vi "Lab_2_subVI_tank_2_Ashish.vi"(0 "H1":dbl, 1 "a1":dbl, 2 "a2":dbl, 3 "A2":dbl, 4 "hss,1":dbl, 5 "hss,2":dbl) -> (14 "H 2":dbl, 15 "h2":dbl)   [LabVIEW 2020]
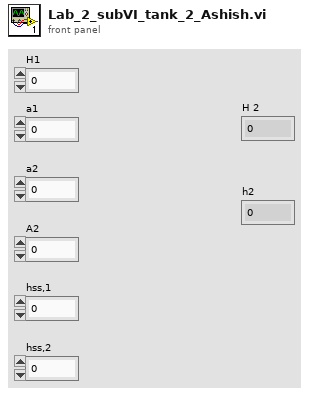
[diagram p1: front panel]
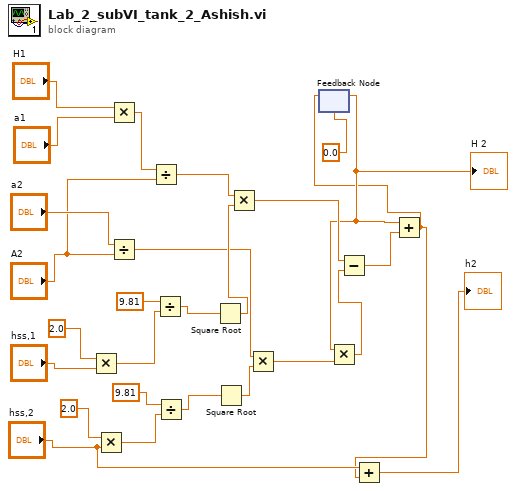
[diagram p0: block diagram]
diagram:
  n1 = Multiply(x=2.0, y="hss,1") -> (x*y=w19:dbl)
  n2 = Multiply(x=2.0, y="hss,2") -> (x*y=w13:dbl)
  n3 = Multiply(x="H1", y="a1") -> (x*y=w24:dbl)
  n4 = Divide(x="a2", y="A2") -> (x/y=w11:dbl)
  n5 = Divide(x=w24, y="A2") -> (x/y=w16:dbl)
  n6 = Divide(x=9.81, y=w19) -> (x/y=w18:dbl)
  n7 = Divide(x=9.81 ("y"), y=w13) -> (x/y=w12:dbl)
  n8 = Square Root(x=w18) -> (sqrt(x)=w17:dbl)
  n9 = Square Root(x=w12) -> (sqrt(x)=w10:dbl)
  n10 = Multiply(x=w16, y=w17) -> (x*y=w9:dbl)
  n11 = Multiply(x=w11, y=w10) -> (x*y=w8:dbl)
  n12 = feedback #1(0.0 ("x-y")) -> (w5:dbl)
  "H 2" <- w5
  n13 = Multiply(x=w5, y=w8) -> (x*y=w7:dbl)
  n14 = Subtract(x=w9, y=w7) -> (x-y=w4:dbl)
  n15 = Add(x=w5, y=w4) -> (x+y=w1:dbl)
  n16 = feedback-in #1(w1) -> ()
  n17 = Add(x="hss,2", y=w1) -> (x+y=→"h2":dbl)
